vi "Control Move Duplicate.vi"(8 "error in":errorcluster, 9 "Owner":refnum<vi>, 10 "Control Array":refnum<vi>[](array[refnum])) -> (0 "error out":errorcluster)   [LabVIEW 2021, in "_Msg Rescript.lvlib" / "_Msg Rescript.lvclass"]
uses:
  _Msg Rescript.lvclass
  _Msg Rescript.lvclass/_Msg Rescript.ctl
  <vilib>/Utility/miscctls.llb/LVPositionTypeDef.ctl
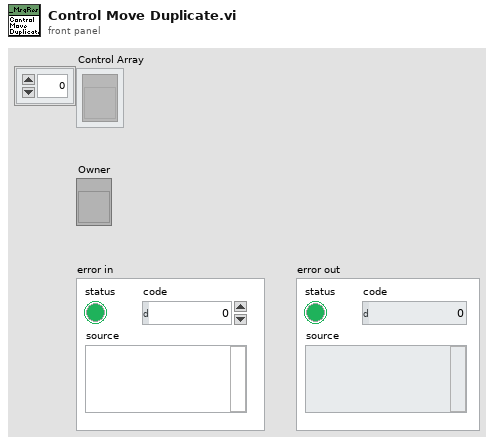
[diagram p1: front panel]
types:
  T1 = typedef "LVPositionTypeDef.ctl" = cluster{"Left":i32, "Top":i32}
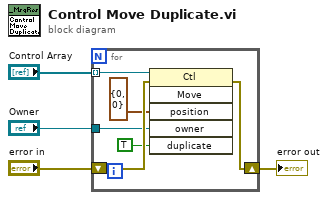
[diagram p0: block diagram]
diagram:
  n1 = for {
    tunnel: "Owner" -> [w9]
    shift-right: [w8] -> w1
    shift-left: "error in" -> [w10]
    tunnel: "Control Array" -> [w7] mode=indexing
    n2 = invoke class="Ctl" method="Move"(reference=w7, error in=w10, "position"=T1 {"Left"=0, "Top"=0}, "owner"=w9, "duplicate"=TRUE ("Duplicate? (F)")) -> (error out=w8:errorcluster)  [unwired: 1 in, 5 out]
  }
  "error out" <- w1
